vi "convert j1939 db to cluster.vi"(8 "error in":errorcluster, 11 "xnet db":refnum<k21>) -> (0 "error out":errorcluster, 3 "system db":T1)   [LabVIEW 2013, in "J1939.lvlib"]
uses:
  J1939.lvlib
  TypeDefs/J1939 db.ctl
  TypeDefs/J1939 db frame.ctl
  TypeDefs/J1939 db signal.ctl
  TypeDefs/J1939 db frame direction.ctl
  Internals/Frame Conversion/Convert CAN Arb ID to J1939 ID.vi
  <vilib>/xnet/xnet.llb/XNET Database Close (Database).vi
  <resource>/objmgr/xnet.rc
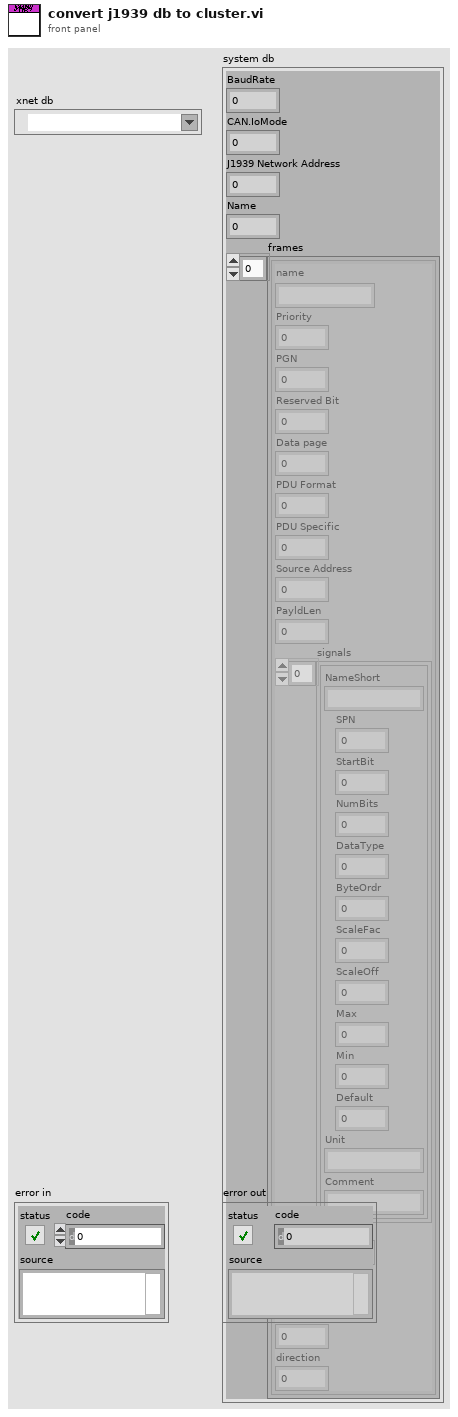
[diagram p1: front panel]
types:
  T1 = typedef "J1939.lvlib/J1939 db.ctl" = cluster{"BaudRate":u32, "CAN.IoMode":u32, "J1939 Network Address":u8, "Name":u64, "frames":T2[]}
  T2 = typedef "J1939.lvlib/J1939 db frame.ctl" = cluster{"name":string, "Priority":u8, "PGN":u32, "Reserved Bit":u8, "Data page":u8, "PDU Format":u8, "PDU Specific":u8, "Source Address":u8, "PayldLen":u32, "signals":T3[], "Comment":string, "can timing type":u32, "transmit time":dbl, "direction":u16}
  T3 = typedef "J1939.lvlib/J1939 db signal.ctl" = cluster{"NameShort":string, "SPN":i32, "StartBit":u32, "NumBits":u32, "DataType":u32, "ByteOrdr":u32, "ScaleFac":dbl, "ScaleOff":dbl, "Max":dbl, "Min":dbl, "Default":dbl, "Unit":string, "Comment":string}
  T4 = typedef "J1939.lvlib/J1939 db frame direction.ctl" = enum16{"Input", "Output", "Input+Output"}
  T5 = typedef "J1939.lvlib/J1939 PGN Fields Cluster.ctl" = cluster{"Reserved Bit":u8, "Data page":u8, "PDU Format":u8, "PDU Specific":u8}
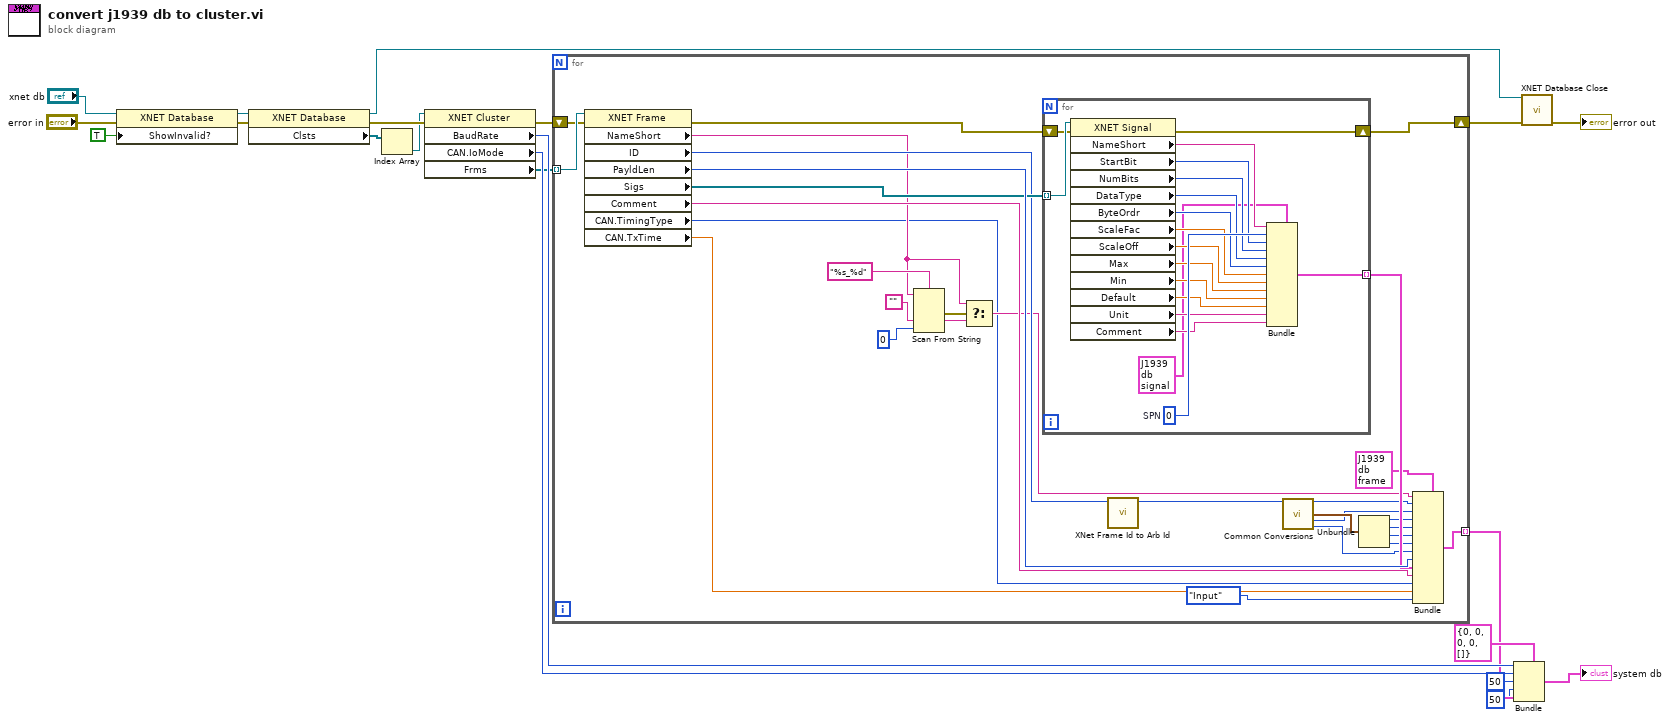
[diagram p0: block diagram]
diagram:
  n1 = property class="XNET Database"(reference="xnet db", error in="error in", "ShowInvalid?"=TRUE ("Show Invalid From Open?")) -> (reference out=w11:refnum<k21>, error out=w12:errorcluster)
  n2 = property class="XNET Database"(reference=w11, error in=w12) -> (reference out=w4:refnum<k21>, error out=w15:errorcluster, "Clsts"=w13:refnum<k21>[])
  n3 = Index Array(array=w13) -> (element=w14:refnum<k21>)  [unwired: 1 in]
  n4 = property class="XNET Cluster"(reference=w14, error in=w15) -> (error out=w7:errorcluster, "BaudRate"=w17:u32, "CAN.IoMode"=w18:u32, "Frms"=w16:refnum<k21>[])  [unwired: 1 out]
  n5 = for {
    tunnel: w16 -> [w50] mode=indexing
    tunnel: [w46] -> w3 mode=indexing
    shift-right: [w32] -> w6
    shift-left: w7 -> [w34]
    n6 = property class="XNET Frame"(reference=w50, error in=w34) -> (error out=w33:errorcluster, "NameShort"=w28:string, "ID"=w36:u32, "PayldLen"=w48:u32, "Sigs"=w47:refnum<k21>[], "Comment"=w37:string, "CAN.TimingType"=w22:u32, "CAN.TxTime"=w23:dbl)  [unwired: 1 out]
    n7 = Scan From String(format string="%s_%d", input string=w28, default 1="", default 2=u8 0 ("default value 1")) -> (error out=w29:errorcluster, output 1=w24:string)  [unwired: 3 in, 2 out]
    n8 = Select(t=w28, s=w29, f=w24) -> (s? t:f=w27:string)
    n9 = for {
      tunnel: w47 -> [w68] mode=indexing
      tunnel: [w54] -> w45 mode=indexing
      shift-right: [w51] -> w32
      shift-left: w33 -> [w52]
      w66 = 0  # SPN
      n10 = property class="XNET Signal"(reference=w68, error in=w52) -> (error out=w51:errorcluster, "NameShort"=w67:string, "StartBit"=w65:u32, "NumBits"=w64:u32, "DataType"=w63:u32, "ByteOrdr"=w62:u32, "ScaleFac"=w61:dbl, "ScaleOff"=w60:dbl, "Max"=w59:dbl, "Min"=w58:dbl, "Default"=w57:dbl, "Unit"=w56:string, "Comment"=w55:string)  [unwired: 1 out]
      n11 = Bundle(cluster=T3 {"NameShort"="", "SPN"=0, "StartBit"=0, "NumBits"=0, "DataType"=0, "ByteOrdr"=0, "ScaleFac"=0.0, "ScaleOff"=0.0, "Max"=0.0, "Min"=0.0, "Default"=0.0, "Unit"="", "Comment"=""} ("output cluster"), "NameShort"=w67, "SPN"=w66, "StartBit"=w65, "NumBits"=w64, "DataType"=w63, "ByteOrdr"=w62, "ScaleFac"=w61, "ScaleOff"=w60, "Max"=w59, "Min"=w58, "Default"=w57, "Unit"=w56, "Comment"=w55) -> (w54:T3)
    }
    n12 = call "XNet Frame Id to Arb Id.vi"("ID"=w36) -> ("Arb id"=w35:u32)  [unwired: 10 in]
    n13 = call-poly "Common Conversions.vi"("Arb ID"=w35) -> ("Priority"=w43:u8, "PGN Fields"=w49:T5, "PGN"=w42:u32, "Source Address"=w31:u8)  [unwired: 11 out]
    n14 = Unbundle(w49) -> ("Reserved Bit"=w41:u8, "Data page"=w40:u8, "PDU Format"=w39:u8, "PDU Specific"=w38:u8)
    n15 = Bundle(cluster=T2 {"name"="", "Priority"=0, "PGN"=0, "Reserved Bit"=0, "Data page"=0, "PDU Format"=0, "PDU Specific"=0, "Source Address"=0, "PayldLen"=0, "signals"=[], "Comment"="", "can timing type"=0, "transmit time"=0.0, "direction"=0} ("output cluster"), "name"=w27, "Priority"=w43, "PGN"=w42, "Reserved Bit"=w41, "Data page"=w40, "PDU Format"=w39, "PDU Specific"=w38, "Source Address"=w31, "PayldLen"=w48, "signals"=w45, "Comment"=w37, "can timing type"=w22, "transmit time"=w23, "direction"=J1939_db_frame_direction."Input" ("Direction")) -> (w46:T2)
  }
  n16 = Bundle(cluster=T1 {"BaudRate"=0, "CAN.IoMode"=0, "J1939 Network Address"=0, "Name"=0, "frames"=[]} ("output cluster"), "BaudRate"=w17, "CAN.IoMode"=w18, "J1939 Network Address"=u8 50, "Name"=u64 50, "frames"=w3) -> (→"system db":T1)
  n17 = call-poly <vilib>:"XNET Database Close.vi"("database in"=w4, "error in (no error)"=w6) -> ("error out"=→"error out":errorcluster)  [unwired: 13 in]
